vi "General VCO.vi"(8 "fs":dbl=0.1, 9 "range":dbl=0.1, 10 "center frequency":dbl=0.05, 11 "X":dbl[](array[numeric])) -> (0 "error":i32, 3 "Y":dbl[](array[numeric]))   [LabVIEW 2014, in "NI_AALBase.lvlib"]
uses:
  NI_AALBase.lvlib
  Ramp Pattern by Samples.vi
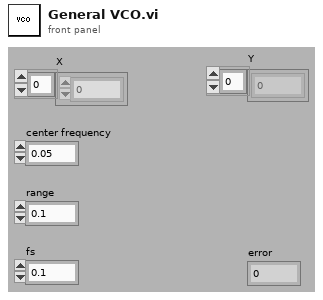
[diagram p1: front panel]
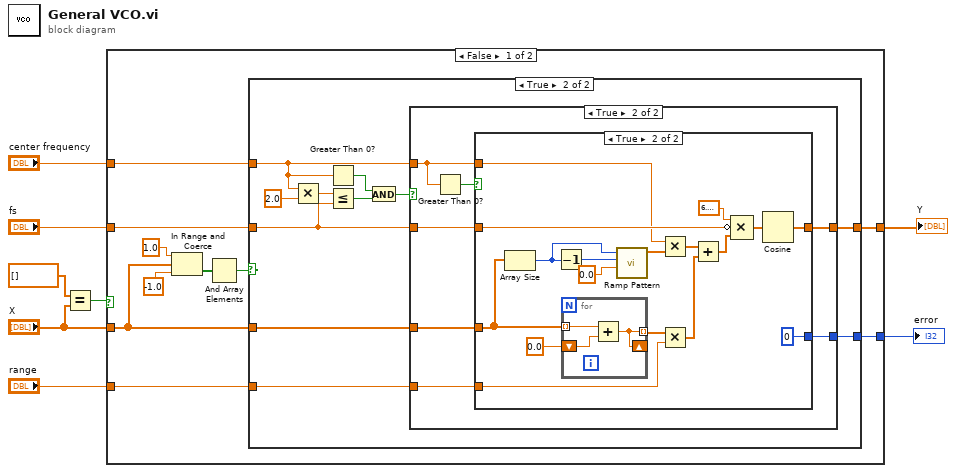
[diagram p0: block diagram]
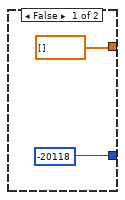
[diagram p2: hidden frame]
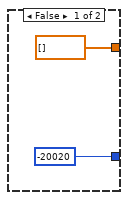
[diagram p3: hidden frame]
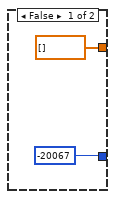
[diagram p4: hidden frame]
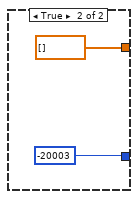
[diagram p5: hidden frame]
diagram:
  n1 = Equal?(x=dbl[] [], y="X") -> (x = y?=w1:bool)
  n2 = case shown="False" w1 {
    tunnel: "center frequency" -> [w16 _]
    tunnel: "fs" -> [w18 _]
    tunnel: [w17 dbl[] []] -> w4
    tunnel: "X" -> [w12 _]
    tunnel: [w10 -20003] -> w8
    tunnel: "range" -> [w9 _]
    frame False {
      n3 = In Range and Coerce(upper limit=1.0, x=w12, lower limit=-1.0) -> (In Range?=w15:bool[])  [unwired: 1 out]
      n4 = And Array Elements(Boolean array=w15) -> (logical AND=w11:bool)
      n5 = case shown="True" w11 {
        tunnel: w18 -> [_ w27]
        tunnel: [dbl[] [] w31] -> w17
        tunnel: w12 -> [_ w30]
        tunnel: w16 -> [_ w25]
        tunnel: [-20118 w26] -> w10
        tunnel: w9 -> [_ w21]
        frame False {
        }
        frame True {
          n6 = Multiply(x=w25, y=2.0) -> (x*y=w29:dbl)
          n7 = Greater Than 0?(x=w25) -> (x > 0?=w24:bool)
          n8 = Less Or Equal?(x=w29, y=w27) -> (x <= y?=w23:bool)
          n9 = And(x=w24, y=w23) -> (x .and. y?=w22:bool)
          n10 = case shown="True" w22 {
            tunnel: w27 -> [_ w40]
            tunnel: [dbl[] [] w39] -> w31
            tunnel: w30 -> [_ w38]
            tunnel: w25 -> [_ w36]
            tunnel: [-20020 w37] -> w26
            tunnel: w21 -> [_ w34]
            frame False {
            }
            frame True {
              n11 = Greater Than 0?(x=w36) -> (x > 0?=w35:bool)
              n12 = case shown="True" w35 {
                tunnel: w40 -> [_ w57]
                tunnel: [dbl[] [] w56] -> w39
                tunnel: w38 -> [_ w54]
                tunnel: w36 -> [_ w46]
                tunnel: [-20067 0] -> w37
                tunnel: w34 -> [_ w48]
                frame False {
                }
                frame True {
                  n13 = Array Size(array=w54) -> (size(s)=w52:i32)
                  n14 = Decrement(x=w52) -> (x-1=w58:i32)
                  n15 = for {
                    tunnel: w54 -> [w62] mode=indexing
                    shift-right: [w60] -> _
                    shift-left: 0.0 -> [w61]
                    tunnel: [w60] -> w49 mode=indexing
                    n16 = Add(x=w62, y=w61) -> (x+y=w60:dbl)
                  }
                  n17 = call-poly "Ramp Pattern.vi"("start"=0.0, "end"=w58, "samples"=w52) -> ("Ramp Pattern"=w51:dbl[])  [unwired: 7 in, 1 out]
                  n18 = Multiply(x=w46, y=w51) -> (x*y=w50:dbl[])
                  n19 = Multiply(x=w49, y=w48) -> (x*y=w47:dbl[])
                  n20 = Add(x=w50, y=w47) -> (x+y=w44:dbl[])
                  n21 = Compound Arithmetic op=MULTIPLY(6.283185307179586, invert w57, w44) -> (w43:dbl[])
                  n22 = Cosine(x=w43) -> (cos(x)=w56:dbl[])
                }
              }
            }
          }
        }
      }
    }
    frame True {
    }
  }
  "error" <- w8
  "Y" <- w4
